vi "FastRoutineSample.vi"() -> ()   [LabVIEW 2014]
doc: "This VI demonstrates how to work with a F-712 system for fast alignment tasks.\nIn the VI menu, several fast alignment settings are accessible as well as axes control tools.\n\nThe diagram shows how to combine the driver VIs for fast alignment tasks. \n\nNote: Run XXXX_Configuration_Setup (with XXXX being the product number of your PI controller) prior to running this VI."
uses:
  C:/ProgramData/PI/LabVIEW/Low Level/General command.llb/Controller names.ctl
  FastRoutineSupportVIs/Message Cluster.ctl
  C:/ProgramData/PI/LabVIEW/Low Level/General command.llb/Global2 (Array).vi
  <vilib>/Utility/file.llb/Write To Spreadsheet File (DBL).vi
panel:
  in  "Clear Error":bool
  in  "Event timeout":i32=40
  out "3DGraphReferenceArray":refnum<vi>[](array[refnum])
  in  "Stop Motion":bool
  out "Area Scan Data":dbl[][][](array[numeric]) format="%.2f"
  out "Gradient Scan Names":string[](array[string])
  out "Analog value":dbl format="%.6f"
  in  "Analog Input":i32=1 min=1 max=10 step=1
  out "Waveform Chart":dbl(graph)
  in  "Routines Tab":T1(tab)
  in  "Area Scan Routines":T3(array[cluster]) {"Sys" min=1 step=1}
  in  "Gradient Scan Routines":T4(array[cluster]) {"Sys" min=1 step=1}
  in  "Start GS Routines":bool
  in  "Stop GS Routines":bool
  out "Controller name":T2
  in  "System no.":i32=1 min=1 step=1
  out "Status Message":string
  in  "Stop":bool
  # "This VI demonstrates how to work with a F-712 system for fast alignment tasks.\nIn the VI menu, several fast alignment settings are accessible as well as axes control tools.\n\nThe diagram shows how to combine the driver VIs for fast alignment tasks. \n\nNote:  Run XXXX_Configuration_Setup (with XXXX being the product number of your PI controller) prior to running this VI."
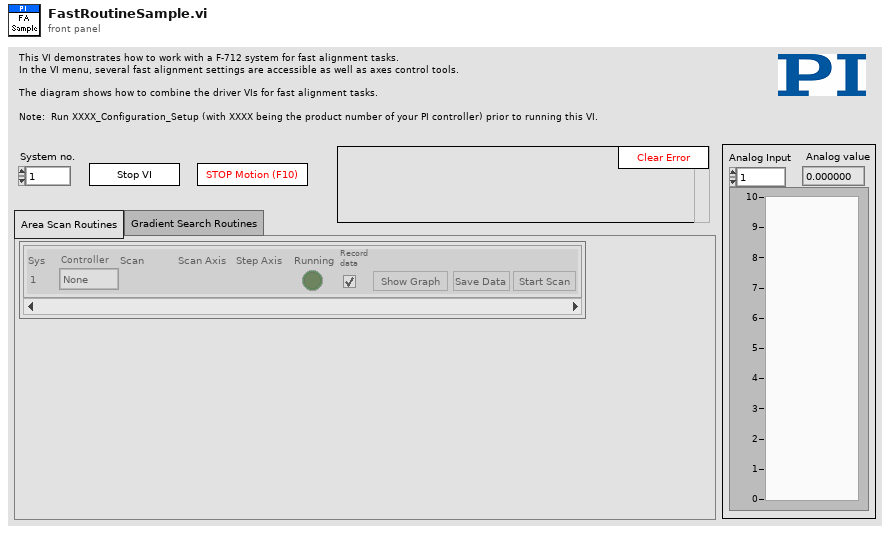
[diagram p1: front panel]
types:
  T1 = enum32{"Area Scan Routines", "Gradient Search Routines"}
  T2 = typedef "Controller names.ctl" = enum16{"None", "Analog", "C-702", "C-413", "C-414", "C-843", "C-843.PM", "C-844", "C-848", "C-865", "C-866", "C-867", "C-877", "C-880", "C-884", "C-885", "C-886", "C-887", "C-891", "E-135", "E-516", "E-517", "E-518", "E-709", "E-710", "E-712", "E-725", "E-727", "E-753", "E-754", "E-755", "E-761", "E-816", "E-861", "E-870", "E-871", "E-872", "E-873", "E-874", "F-206", "HydraPollux", "M-840", "M-850", "M-8X0", "Mercury", "Mercury_GCS", "PI_GCS2"}
  T3 = cluster{"Sys":i32, "Controller":T2, "Scan":string, "Scan Axis":string, "Step Axis":string, "Running":bool, "Record\ndata":bool, "Show Graph":bool, "Save Data":bool, "Start Scan":bool}[]
  T4 = cluster{"Sys":i32, "Scan":string, "Scan Axis":string, "Step Axis":string, "Running":bool, "Enable":bool, "Show Graph":bool, "Controller":T2, "Show Raw Data":bool}[]
  T5 = typedef "Message Cluster.ctl" = cluster{"Message":string, "Message Data":variant}
  T6 = cluster{"Sys":i32, "Scan":string, "Scan Axis":string, "Step Axis":string, "Running":bool, "Enable":bool, "Show Graph":bool, "Controller":T2, "Show Raw Data":bool}
  T7 = cluster{"Sys":i32, "Controller":T2, "Scan":string, "Scan Axis":string, "Step Axis":string, "Running":bool, "Record\ndata":bool, "Show Graph":bool, "Save Data":bool, "Start Scan":bool}
  T8 = cluster{"System No.":i32, "Scan":string, "Scan Axis":string, "Step Axis":string, "Running":bool, "Enable":bool, "Show Graph":bool, "Controller":T2, "Show Raw Data":bool}
  T9 = enum16{"open", "replace", "create", "open or create", "replace or create", "replace or create with confirmation"}
  T10 = cluster{"Gradient Scan Names":string[], "Dither Radius":dbl[], "Scan axis center":dbl[], "Step axis center":dbl[]}
  T11 = cluster{"Axis":string, "Target":dbl, "System no.":i32}
  T12 = cluster{"String to send":string, "System no.":i32}
  T13 = cluster{"Conn. axes":string[], "Controller name":T2}[]
  T14 = cluster{"Conn. axes":string[], "Controller name":T2}
  T15 = cluster{"Scan name":string, "Scan range minimum":dbl, "Scan range maximum":dbl, "Step range minimum":dbl, "Step range maximum":dbl}[]
  T16 = cluster{"Sys":i32, "Controller":T2, "Scan":string, "Successful":bool, "Signal Intensity at max":dbl, "Positions at max.":string, "Duration (s)":dbl}[]
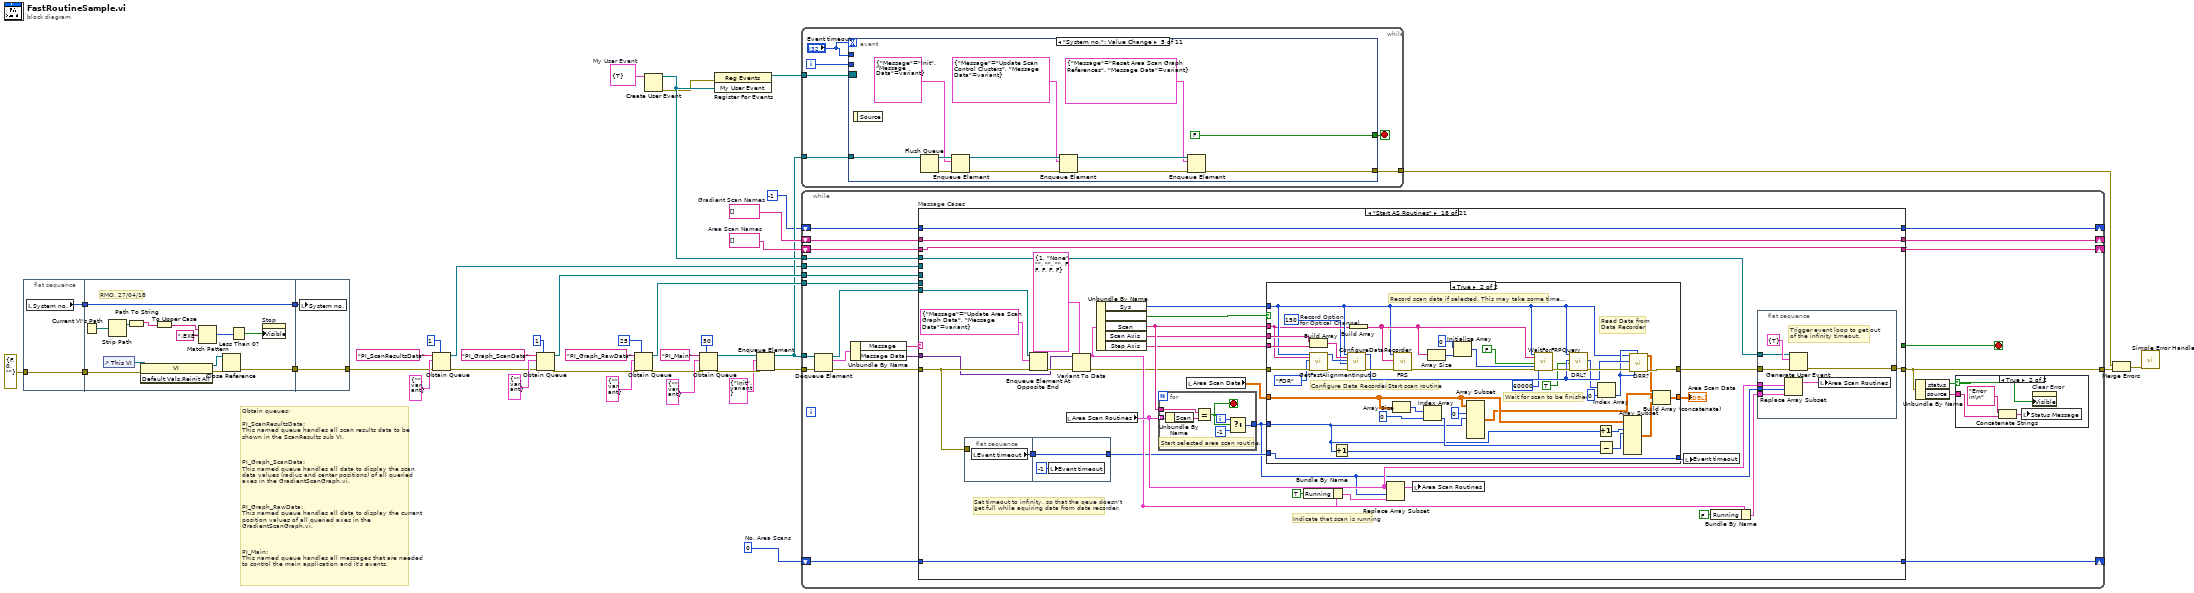
[diagram p0: block diagram]
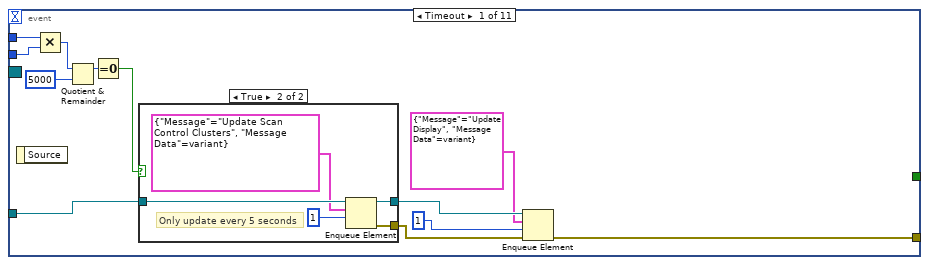
[diagram p2: hidden frame]
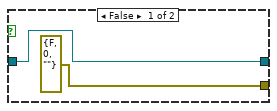
[diagram p3: hidden frame]
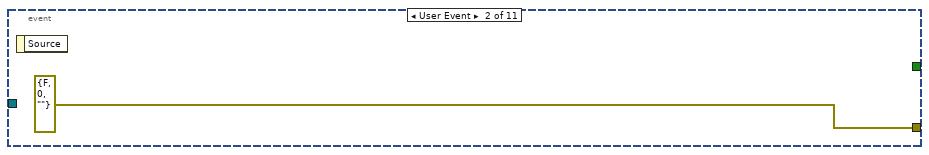
[diagram p4: hidden frame]
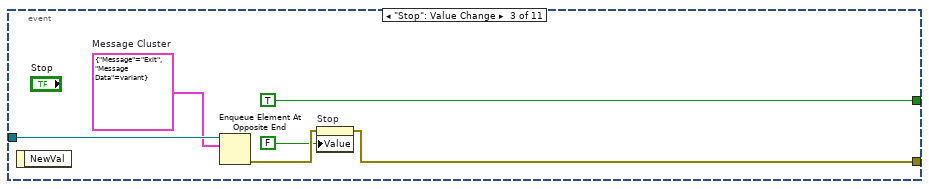
[diagram p5: hidden frame]
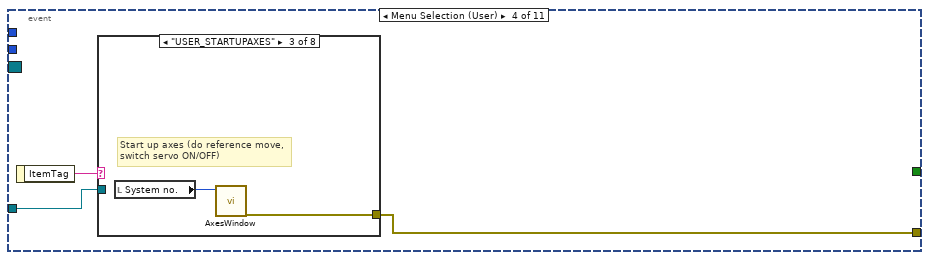
[diagram p6: hidden frame]
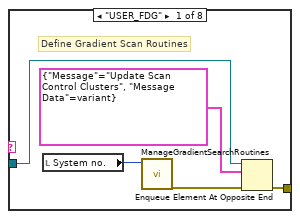
[diagram p7: hidden frame]
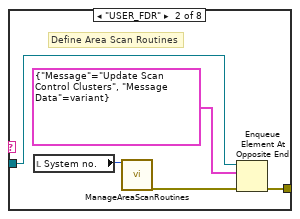
[diagram p8: hidden frame]
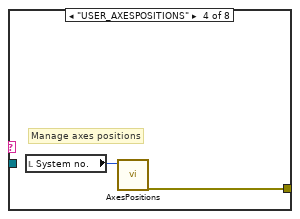
[diagram p9: hidden frame]
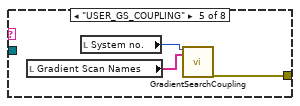
[diagram p10: hidden frame]
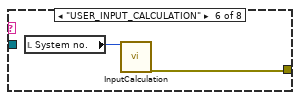
[diagram p11: hidden frame]
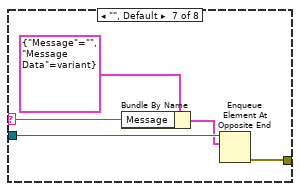
[diagram p12: hidden frame]
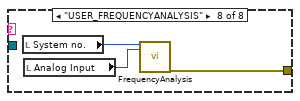
[diagram p13: hidden frame]
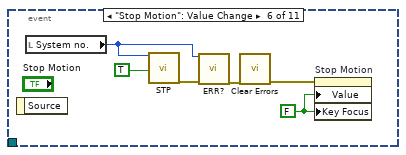
[diagram p14: hidden frame]
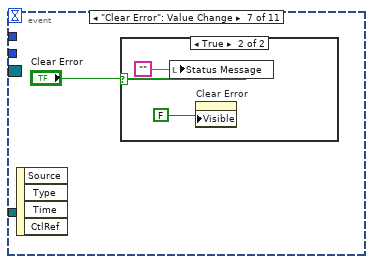
[diagram p15: hidden frame]
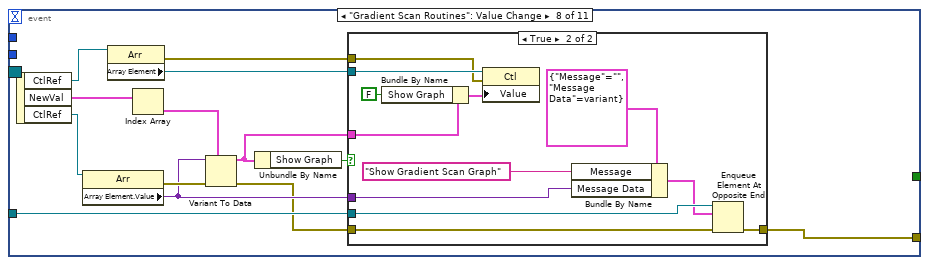
[diagram p17: hidden frame]
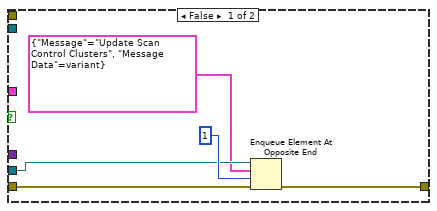
[diagram p18: hidden frame]
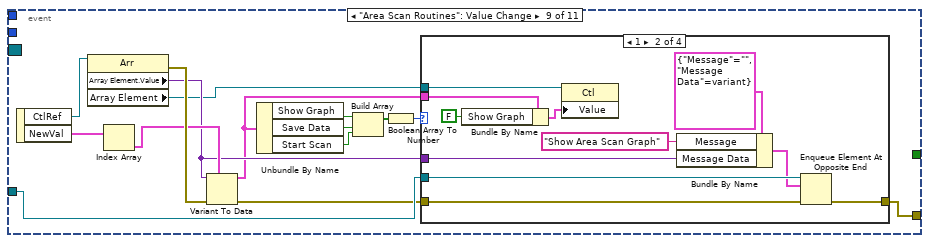
[diagram p19: hidden frame]
diagram:
  w8 = cluster{"Trigger":bool} {"Trigger"=TRUE}  # My User Event
  w20 = 0  # No. Area Scans
  w22 = string[] []  # Area Scan Names
  w23 = string[] []  # Gradient Scan Names
  # "Obtain queues:\n\nPI_ScanResultsData:\nThis named queue handles all scan results data to be shown in the ScanResults sub VI.\n\n\n\nPI_Graph_ScanData:\nThis named queue handles all data to display the scan data values (radius and center positions) of all queried axes in the GradientScanGraph.vi. \n\n\n\nPI_Graph_RawData:\nThis named queue handles all data to display the current position values of all queried axes in the GradientScanGraph.vi. \n\n\n\nPI_Main:\nThis named queue handles all messages that are needed to control the main application and it's events."
  n1 = flat-sequence {
    tunnel: errorcluster {"status"=FALSE, "code"=0, "source"=""} ("error in (no error)") -> [w42]
    tunnel: [w42] -> w3
    tunnel: [w41] -> w1
    tunnel: [w52] -> w4
    tunnel: w3 -> [w51]
    tunnel: [w50] -> w2
    tunnel: w1 -> [w50]
    tunnel: [w57] -> w11
    tunnel: w4 -> [w57]
    tunnel: w2 -> [w56]
    frame #0 {
      n2 = local read "System no."() -> (w41:i32)
    }
    frame #1 {
      # "RMO, 27/04/18"
      n3 = Current VI's Path() -> (path=w44:path)
      n4 = control-ref of="This VI"() -> (w55:refnum<vi>)
      n5 = Strip Path(path=w44) -> (stripped path=w45:path)  [unwired: 1 out]
      n6 = Path To String(path=w45) -> (string=w46:string)
      n7 = invoke class="VI" method="Default Vals.Reinit All"(reference=w55, error in=w51) -> (reference out=w54:refnum<vi>, error out=w53:errorcluster)  [unwired: 1 in, 1 out]
      n8 = To Upper Case(1:w46) -> (0:w47:string)
      n9 = Match Pattern(string=w47, regular expression=".EXE") -> (offset past match=w49:i32)  [unwired: 4 out]
      n10 = Close Reference(reference=w54, error in (no error)=w53) -> (error out=w52:errorcluster)
      n11 = Less Than 0?(x=w49) -> (x < 0?=w43:bool)
      n12 = property on="Stop" class="Bool (strict)"("Visible"=w43) -> ()  [unwired: 2 in, 2 out]
    }
    frame #2 {
      n13 = local write "System no."(w56) -> ()
    }
  }
  n14 = Obtain Queue(max queue size (-1, unlimited)=1, name (unnamed)="PI_ScanResultsData", element data type=T5 {"Message"="", "Message Data"=variant} ("Message Cluster"), error in (no error)=w11) -> (queue out=w10:refnum<queue>, error out=w12:errorcluster)  [unwired: 1 in, 1 out]
  n15 = Obtain Queue(max queue size (-1, unlimited)=1, name (unnamed)="PI_Graph_ScanData", element data type=T5 {"Message"="", "Message Data"=variant} ("Message Cluster"), error in (no error)=w12) -> (queue out=w24:refnum<queue>, error out=w25:errorcluster)  [unwired: 1 in, 1 out]
  n16 = Obtain Queue(max queue size (-1, unlimited)=25, name (unnamed)="PI_Graph_RawData", element data type=T5 {"Message"="", "Message Data"=variant} ("Message Cluster"), error in (no error)=w25) -> (queue out=w30:refnum<queue>, error out=w19:errorcluster)  [unwired: 1 in, 1 out]
  n17 = Create User Event(user event datatype=w8) -> (user event=w40:refnum<user-event>, error out=w9:errorcluster)  [unwired: 1 in]
  n18 = Obtain Queue(max queue size (-1, unlimited)=50, name (unnamed)="PI_Main", element data type=T5 {"Message"="", "Message Data"=variant} ("Message Cluster"), error in (no error)=w19) -> (queue out=w37:refnum<queue>, error out=w38:errorcluster)  [unwired: 1 in, 1 out]
  n19 = register-events(error in=w9, w40) -> (reference out=w7:refnum<event-registration>)  [unwired: 1 in, 1 out]
  n20 = Enqueue Element(queue=w37, element=T5 {"Message"="Init", "Message Data"=variant}, error in (no error)=w38) -> (queue out=w21:refnum<queue>, error out=w36:errorcluster)  [unwired: 2 out]
  n21 = while {
    tunnel: w21 -> [w63]
    tunnel: [w61] -> w18
    tunnel: w7 -> [w59]
    i -> [w60]
    stop <- w62 stop-if-true
    n22 = event shown="[4] \"System no.\": Value Change" {
      selector: w59 -> [_ _ _ _ _ _ _ _ _ _ _]
      dyn-events: _ -> [_ _ _ _ _ _ _ _ _ _ _]
      timeout: "Event timeout" -> [_ _ _ _ _ _ _ _ _ _ _]
      tunnel: [_ _ TRUE _ FALSE _ _ _ _ _ _] -> w62
      tunnel: w63 -> [w68 _ w89 w90 w130 _ _ w153 w185 w224 w231]
      tunnel: [w71 errorcluster {"status"=FALSE, "code"=0, "source"=""} ("error out") w86 w91 w123 _ _ w152 w184 w225 w226] -> w61
      tunnel: w60 -> [w66 _ _ _ _ _ _ _ _ _ _]
      tunnel: "Event timeout" -> [w67 _ _ _ _ _ _ _ _ _ _]
      event Timeout {
        n23 = event-data() -> ()  [unwired: 2 out]
        n24 = Multiply(x=w67, y=w66) -> (x*y=w65:i32)
        n25 = Quotient & Remainder(x=w65, y=5000) -> (x-y*floor(x/y)=w74:i32)  [unwired: 1 out]
        n26 = Equal To 0?(x=w74) -> (x = 0?=w73:bool)
        n27 = case shown="True" w73 {
          tunnel: [errorcluster {"status"=FALSE, "code"=0, "source"=""} ("error out") w82] -> w70
          tunnel: w68 -> [w76 w81]
          tunnel: [w76 w79] -> w69
          frame False {
          }
          frame True {
            # "Only update every 5 seconds"
            n28 = Enqueue Element(queue=w81, element=T5 {"Message"="Update Scan Control Clusters", "Message Data"=variant} ("Message Cluster"), timeout in ms (-1)=1) -> (queue out=w79:refnum<queue>, error out=w82:errorcluster)  [unwired: 1 in, 1 out]
          }
        }
        n29 = Enqueue Element(queue=w69, element=T5 {"Message"="Update Display", "Message Data"=variant} ("Message"), timeout in ms (-1)=1, error in (no error)=w70) -> (error out=w71:errorcluster)  [unwired: 2 out]
      }
      event User Event {
        n30 = event-data() -> ()  [unwired: 2 out]
      }
      event "Stop": Value Change {
        w84 = T5 {"Message"="Exit", "Message Data"=variant}  # Message Cluster
        n31 = event-data() -> ()  [unwired: 2 out]
        n32 = Enqueue Element At Opposite End(queue=w89, element=w84) -> (error out=w87:errorcluster)  [unwired: 1 in, 3 out]
        n33 = property on="Stop" class="Bool (strict)"(error in=w87, "Value"=FALSE) -> (error out=w86:errorcluster)  [unwired: 1 in, 1 out]
      }
      event Menu Selection (User) {
        n34 = event-data() -> ("ItemTag"=w92:string)  [unwired: 1 out]
        n35 = case shown="\"USER_STARTUPAXES\"" w92 {
          selector: w92 -> [_ _ _ _ _ _ w113 _]
          tunnel: [w96 w99 w104 w106 w109 w111 w116 w119] -> w91
          tunnel: w90 -> [w95 w100 _ _ _ _ w115 _]
          frame "USER_FDG" {
            # "Define Gradient Scan Routines"
            n36 = local read "System no."() -> (w93:i32)
            n37 = call "ManageGradientSearchRoutines.vi"("System no."=w93) -> ("error out"=w97:errorcluster)  [unwired: 1 in, 17 out]
            n38 = Enqueue Element At Opposite End(queue=w95, element=T5 {"Message"="Update Scan Control Clusters", "Message Data"=variant} ("Message Cluster"), error in (no error)=w97) -> (error out=w96:errorcluster)  [unwired: 3 out]
          }
          frame "USER_FDR" {
            # "Define Area Scan Routines"
            n39 = local read "System no."() -> (w98:i32)
            n40 = call "ManageAreaScanRoutines.vi"("System no."=w98) -> ("error out"=w101:errorcluster)  [unwired: 1 in, 17 out]
            n41 = Enqueue Element At Opposite End(queue=w100, element=T5 {"Message"="Update Scan Control Clusters", "Message Data"=variant} ("Message Cluster"), error in (no error)=w101) -> (error out=w99:errorcluster)  [unwired: 3 out]
          }
          frame "USER_STARTUPAXES" {
            # "Start up axes (do reference move, \nswitch servo ON/OFF)"
            n42 = local read "System no."() -> (w103:i32)
            n43 = call "AxesWindow.vi"("System no."=w103) -> ("error out"=w104:errorcluster)  [unwired: 1 in, 17 out]
          }
          frame "USER_AXESPOSITIONS" {
            # "Manage axes positions"
            n44 = local read "System no."() -> (w105:i32)
            n45 = call "AxesPositions.vi"("System no."=w105) -> ("error out"=w106:errorcluster)  [unwired: 1 in, 17 out]
          }
          frame "USER_GS_COUPLING" {
            n46 = local read "Gradient Scan Names"() -> (w108:string[])
            n47 = local read "System no."() -> (w107:i32)
            n48 = call "GradientSearchCoupling.vi"("System no."=w107, "Gradient Scan Names"=w108) -> ("error out"=w109:errorcluster)  [unwired: 1 in, 16 out]
          }
          frame "USER_INPUT_CALCULATION" {
            n49 = local read "System no."() -> (w110:i32)
            n50 = call "InputCalculation.vi"("System no."=w110) -> ("error out"=w111:errorcluster)  [unwired: 1 in, 17 out]
          }
          frame "", Default {
            n51 = Bundle By Name(cluster=T5 {"Message"="", "Message Data"=variant} ("Message"), "Message"=w113) -> (w112:T5)
            n52 = Enqueue Element At Opposite End(queue=w115, element=w112) -> (error out=w116:errorcluster)  [unwired: 1 in, 3 out]
          }
          frame "USER_FREQUENCYANALYSIS" {
            n53 = local read "System no."() -> (w118:i32)
            n54 = local read "Analog Input"() -> (w117:i32)
            n55 = call "FrequencyAnalysis.vi"("System no."=w118, "Analog Input Channel"=w117) -> ("error out"=w119:errorcluster)  [unwired: 1 in, 16 out]
          }
        }
      }
      event "System no.": Value Change {
        n56 = event-data() -> ()  [unwired: 2 out]
        n57 = Flush Queue(queue=w130) -> (queue out=w128:refnum<queue>, error out=w129:errorcluster)  [unwired: 1 in, 1 out]
        n58 = Enqueue Element(queue=w128, element=T5 {"Message"="Init", "Message Data"=variant} ("Message"), error in (no error)=w129) -> (queue out=w127:refnum<queue>, error out=w126:errorcluster)  [unwired: 2 out]
        n59 = Enqueue Element(queue=w127, element=T5 {"Message"="Update Scan Control Clusters", "Message Data"=variant} ("Message"), error in (no error)=w126) -> (queue out=w124:refnum<queue>, error out=w125:errorcluster)  [unwired: 2 out]
        n60 = Enqueue Element(queue=w124, element=T5 {"Message"="Reset Area Scan Graph References", "Message Data"=variant} ("Message"), error in (no error)=w125) -> (error out=w123:errorcluster)  [unwired: 3 out]
      }
      event "Stop Motion": Value Change {
        w132 = FALSE
        n61 = event-data() -> ()  [unwired: 2 out]
        n62 = local read "System no."() -> (w135:i32)
        n63 = call "STP.vi"("System no."=w135, "All axes?"=TRUE) -> ("error out"=w136:errorcluster)  [unwired: 3 in, 14 out]
        n64 = call "ERR?.vi"("System no."=w135, "error in"=w136) -> ("error out"=w134:errorcluster)  [unwired: 17 out]
        n65 = call <vilib>:"Clear Errors.vi"("error in (no error)"=w134) -> ("error out"=w133:errorcluster)  [unwired: 1 in, 5 out]
        n66 = property on="Stop Motion" class="Bool"(error in=w133, "Value"=w132, "Key Focus"=w132) -> ()  [unwired: 1 in, 2 out]
      }
      event "Clear Error": Value Change {
        n67 = event-data() -> ()  [unwired: 5 out]
        n68 = case shown="True" "Clear Error" {
          frame False {
          }
          frame True {
            n69 = local write "Status Message"("") -> ()
            n70 = property on="Clear Error" class="Bool"("Visible"=FALSE) -> ()  [unwired: 2 in, 2 out]
          }
        }
      }
      event "Gradient Scan Routines": Value Change {
        n71 = event-data() -> ("CtlRef"=w143:refnum<vi>, "NewVal"=w149:T4, "CtlRef"=w144:refnum<vi>)  [unwired: 1 out]
        n72 = property class="Arr"(reference=w144) -> (error out=w151:errorcluster, "Array Element.Value"=w148:variant)  [unwired: 1 in, 1 out]
        n73 = property class="Arr"(reference=w143) -> (error out=w141:errorcluster, "Array Element"=w142:refnum<vi>)  [unwired: 1 in, 1 out]
        n74 = Index Array(array=w149) -> (element=w150:T6)  [unwired: 1 in]
        n75 = Variant To Data(error in=w151, type=w150, Variant=w148) -> (data=w145:T6, error out=w147:errorcluster)
        n76 = Unbundle By Name(w145) -> ("Show Graph"=w146:bool)
        n77 = case shown="True" w146 {
          tunnel: w153 -> [w155 w170]
          tunnel: [w156 w169] -> w152
          tunnel: w148 -> [_ w166]
          tunnel: w147 -> [w157 w165]
          tunnel: w142 -> [_ w162]
          tunnel: w145 -> [_ w161]
          tunnel: w141 -> [_ w159]
          frame False {
            n78 = Enqueue Element At Opposite End(queue=w155, element=T5 {"Message"="Update Scan Control Clusters", "Message Data"=variant} ("Message"), timeout in ms (-1)=1, error in (no error)=w157) -> (error out=w156:errorcluster)  [unwired: 2 out]
          }
          frame True {
            n79 = Bundle By Name(cluster=w161, "Show Graph"=FALSE) -> (w163:T6)
            n80 = property class="Ctl"(reference=w162, error in=w159, "Value"=w163) -> ()  [unwired: 2 out]
            n81 = Bundle By Name(cluster=T5 {"Message"="", "Message Data"=variant} ("Message"), "Message"="Show Gradient Scan Graph", "Message Data"=w166) -> (w168:T5)
            n82 = Enqueue Element At Opposite End(queue=w170, element=w168, error in (no error)=w165) -> (error out=w169:errorcluster)  [unwired: 3 out]
          }
        }
      }
      event "Area Scan Routines": Value Change {
        n83 = event-data() -> ("CtlRef"=w171:refnum<vi>, "NewVal"=w177:T3)  [unwired: 1 out]
        n84 = property class="Arr"(reference=w171) -> (error out=w183:errorcluster, "Array Element.Value"=w181:variant, "Array Element"=w179:refnum<vi>)  [unwired: 1 in, 1 out]
        n85 = Index Array(array=w177) -> (element=w182:T7)  [unwired: 1 in]
        n86 = Variant To Data(error in=w183, type=w182, Variant=w181) -> (data=w178:T7, error out=w180:errorcluster)
        n87 = Unbundle By Name(w178) -> ("Show Graph"=w176:bool, "Save Data"=w175:bool, "Start Scan"=w172:bool)
        n88 = Build Array(w176, w175, w172) -> (w174:bool[])
        n89 = Boolean Array To Number(Boolean array=w174) -> (number=w173:u32)
        n90 = case shown="1" w173 {
          tunnel: w185 -> [_ w197 w208 w219]
          tunnel: [w186 w196 w207 w218] -> w184
          tunnel: w181 -> [_ w193 w199 _]
          tunnel: w180 -> [w186 w192 w204 w211]
          tunnel: w179 -> [_ w189 w201 w213]
          tunnel: w178 -> [_ w188 w200 w212]
          frame 0, Default {
          }
          frame 1 {
            n91 = Bundle By Name(cluster=w188, "Show Graph"=FALSE) -> (w190:T7)
            n92 = property class="Ctl"(reference=w189, "Value"=w190) -> ()  [unwired: 1 in, 2 out]
            n93 = Bundle By Name(cluster=T5 {"Message"="", "Message Data"=variant} ("Message"), "Message"="Show Area Scan Graph", "Message Data"=w193) -> (w195:T5)
            n94 = Enqueue Element At Opposite End(queue=w197, element=w195, error in (no error)=w192) -> (error out=w196:errorcluster)  [unwired: 3 out]
          }
          frame 2 {
            n95 = Bundle By Name(cluster=w200, "Save Data"=FALSE) -> (w202:T7)
            n96 = property class="Ctl"(reference=w201, "Value"=w202) -> ()  [unwired: 1 in, 2 out]
            n97 = Bundle By Name(cluster=T5 {"Message"="", "Message Data"=variant} ("Message"), "Message"="Save Area Scan Data", "Message Data"=w199) -> (w206:T5)
            n98 = Enqueue Element At Opposite End(queue=w208, element=w206, error in (no error)=w204) -> (error out=w207:errorcluster)  [unwired: 3 out]
          }
          frame 4 {
            n99 = Bundle By Name(cluster=w212, "Start Scan"=FALSE) -> (w214:T7)
            n100 = property class="Ctl"(reference=w213, "Value"=w214) -> ("Value"=w209:variant)  [unwired: 1 in, 2 out]
            n101 = Bundle By Name(cluster=T5 {"Message"="", "Message Data"=variant} ("Message"), "Message"="Start AS Routines", "Message Data"=w209) -> (w217:T5)
            n102 = Enqueue Element At Opposite End(queue=w219, element=w217, error in (no error)=w211) -> (error out=w218:errorcluster)  [unwired: 3 out]
          }
        }
      }
      event "Start GS Routines": Value Change {
        w220 = T5 {"Message"="", "Message Data"=variant}  # Message Cluster
        n103 = event-data() -> ("CtlRef"=w223:refnum<vi>)  [unwired: 1 out]
        n104 = property class="Bool"(reference=w223) -> ("Label.Text"=w222:string)  [unwired: 1 in, 2 out]
        n105 = Bundle By Name(cluster=w220, "Message"=w222) -> (w221:T5)
        n106 = Enqueue Element At Opposite End(queue=w224, element=w221) -> (error out=w225:errorcluster)  [unwired: 1 in, 3 out]
      }
      event "Stop GS Routines": Value Change {
        w227 = T5 {"Message"="", "Message Data"=variant}  # Message Cluster
        n107 = event-data() -> ("CtlRef"=w230:refnum<vi>)  [unwired: 1 out]
        n108 = property class="Bool"(reference=w230) -> ("Label.Text"=w229:string)  [unwired: 1 in, 2 out]
        n109 = Bundle By Name(cluster=w227, "Message"=w229) -> (w228:T5)
        n110 = Enqueue Element At Opposite End(queue=w231, element=w228) -> (error out=w226:errorcluster)  [unwired: 1 in, 3 out]
      }
    }
  }
  n111 = while {
    tunnel: w21 -> [w252]
    tunnel: w30 -> [w246]
    tunnel: w24 -> [w245]
    shift-right: [w244] -> _
    shift-left: w23 -> [w243]
    shift-right: [w241] -> _
    shift-left: w22 -> [w242]
    shift-right: [w240] -> _
    shift-left: -1 ("System no.") -> [w239]
    shift-right: [w237] -> _
    shift-left: w20 -> [w238]
    tunnel: w10 -> [w236]
    tunnel: w36 -> [w253]
    tunnel: [w235] -> w17
    tunnel: w40 -> [w232]
    stop <- w254 stop-if-true
    n112 = Dequeue Element(queue=w252, error in (no error)=w253) -> (queue out=w250:refnum<queue>, element=w251:T5, error out=w249:errorcluster)  [unwired: 2 out]
    n113 = Unbundle By Name(w251) -> ("Message"=w248:string, "Message Data"=w247:variant)
    n114 = case "Message Cases" shown="\"Start AS Routines\"" w248 {
      tunnel: w250 -> [w261 _ _ _ _ _ _ _ w608 _ _ w732 _ _ _ w890 _ w960 _ w1083 _]
      tunnel: w249 -> [w272 w308 w324 w354 w418 w485 w517 w567 w612 w630 w665 w750 w815 w873 w887 w902 w925 w961 w1051 w1082 w1094]
      tunnel: [w263 w305 w323 w352 w421 w461 w509 w555 w607 w631 w666 w753 w817 w861 w876 w891 w925 w938 w1052 w1068 w1094] -> w235
      tunnel: [w262 _ _ _ _ _ _ _ _ _ _ _ _ _ _ _ _ _ _ TRUE _] -> w254
      tunnel: w247 -> [_ _ _ _ w419 w484 w516 w566 _ _ _ _ w813 w871 w886 _ _ w958 _ _ _]
      tunnel: w246 -> [_ _ _ _ _ _ _ _ _ _ _ w760 _ _ _ _ _ _ _ _ _]
      tunnel: w245 -> [_ _ _ _ _ _ _ _ _ _ _ w721 _ _ _ _ _ _ _ w1073 _]
      tunnel: [w270 w316 w335 w381 w397 w489 w505 w572 w616 w635 w661 w718 w810 w869 w884 w900 w929 w968 w1046 w1078 w1093] -> w244
      tunnel: w243 -> [_ w316 w335 w381 w397 w489 w505 w572 w616 w635 _ w718 w810 w869 w884 w900 w929 w968 w1046 w1078 w1093]
      tunnel: w242 -> [_ w315 w334 w380 w396 w486 w518 w571 w606 w634 _ w729 w809 w868 w883 w899 w928 w967 w1045 w1077 w1092]
      tunnel: [w271 w315 w334 w380 w396 w486 w518 w571 w606 w634 w675 w729 w809 w868 w883 w899 w928 w967 w1045 w1077 w1092] -> w241
      tunnel: ["System no." w314 w333 w353 w395 w488 w520 w556 w615 w628 w660 w731 w808 w867 w879 w898 w927 w954 w1044 w1076 w1091] -> w240
      tunnel: w239 -> [w260 w314 w333 w353 w395 w488 w520 w556 w615 w628 w660 w731 w808 w867 w879 w898 w927 w954 w1044 w1076 w1091]
      tunnel: w238 -> [w275 w313 w332 w379 w394 w479 w515 w570 _ w633 w676 w733 w801 w864 w882 w896 w926 w964 w1042 w1075 w1090]
      tunnel: [w275 w313 w332 w379 w394 w479 w515 w570 w614 w633 w676 w734 w801 w864 w882 w896 w926 w964 w1042 w1075 w1090] -> w237
      tunnel: w236 -> [_ _ _ _ _ _ _ _ _ _ _ w726 _ _ _ _ _ _ _ w1070 _]
      tunnel: w232 -> [_ _ _ _ _ _ _ _ _ _ _ _ _ _ _ _ _ w942 _ _ _]
      frame "Init" {
        w271 = string[] []  # Area Scan Names
        w270 = string[] []  # Gradient Scan Names
        w259 = "Connected to:\n"
        # "Query identification of connected controller."
        n115 = call "*IDN?.vi"("System no."="System no.", "error in"=w272) -> ("Identification"=w274:string, "error out"=w264:errorcluster)  [unwired: 16 out]
        n116 = Concatenate Strings(w259, w274) -> (→"Status Message":string)
        n117 = call "ERR?.vi"("error in"=w264) -> ("Controller error"=w267:bool, "error out"=w269:errorcluster)  [unwired: 1 in, 16 out]
        n118 = Unbundle By Name(w269) -> ("status"=w268:bool)
        n119 = Not(x=w267) -> (.not. x?=w266:bool)
        n120 = And(x=w266, y=w268) -> (x .and. y?=w265:bool)
        n121 = case shown="True" w265 {
          tunnel: [w282 w290] -> w263
          tunnel: w261 -> [w281 w291]
          tunnel: [FALSE w292] -> w262
          tunnel: w260 -> [_ w287]
          tunnel: w269 -> [w279 w285]
          tunnel: w259 -> [_ w283]
          frame False {
            n122 = call <vilib>:"Clear Errors.vi"("error in (no error)"=w279) -> ("error out"=w278:errorcluster)  [unwired: 1 in, 5 out]
            n123 = Enqueue Element At Opposite End(queue=w281, element=T5 {"Message"="Show ScanResults Window", "Message Data"=variant} ("Message Cluster"), error in (no error)=w278) -> (error out=w282:errorcluster)  [unwired: 3 out]
          }
          frame True {
            n124 = call <vilib>:"Clear Errors.vi"("error in (no error)"=w285) -> ("error out"=w289:errorcluster)  [unwired: 1 in, 5 out]
            n125 = call "*IDN?.vi"("System no."=w287, "error in"=w289) -> ("Identification"=w286:string, "error out"=w284:errorcluster)  [unwired: 16 out]
            n126 = Concatenate Strings(w283, w286) -> (w288:string)
            n127 = local write "Status Message"(w288) -> ()
            n128 = case shown="Error" w284 {
              selector: w284 -> [w294 w297]
              tunnel: [FALSE TRUE] -> w292
              tunnel: w291 -> [_ w303]
              tunnel: [w293 w299] -> w290
              tunnel: w287 -> [w295 _]
              frame No Error {
                # "If previous system number works, \nthen switch back to previous number."
                n129 = property on="System no." class="DigNum (strict)"(error in=w294, "Val(Sgnl)"=w295, "Value"=w295) -> (error out=w293:errorcluster)  [unwired: 1 in, 1 out]
              }
              frame Error {
                # "If *IDN? reports an error,\nthe system is probably not connected."
                n130 = property on="Stop" class="Bool (strict)"("Val(Sgnl)"=TRUE) -> (error out=w300:errorcluster)  [unwired: 2 in, 1 out]
                n131 = Enqueue Element At Opposite End(queue=w303, element=T5 {"Message"="Exit", "Message Data"=variant}, error in (no error)=w300) -> (error out=w298:errorcluster)  [unwired: 3 out]
                n132 = Merge Errors(w297, w298) -> (w299:errorcluster)
              }
            }
          }
        }
      }
      frame "USER_AXESCONTROL" {
        # "Show Axes Control window."
        n133 = vi-ref "AxesControl.vi"() -> (w318:refnum<vi>)
        n134 = property class="VI"(reference=w318, error in=w308) -> (error out=w307:errorcluster, "Path"=w319:path)  [unwired: 1 out]
        n135 = Open VI Reference(vi path=w319, options=8, error in (no error)=w307) -> (vi reference=w317:refnum<vi>, error out=w306:errorcluster)  [unwired: 1 in, 2 out]
        n136 = property class="VI"(reference=w317, error in=w306, "Front Panel.Open"=TRUE ("Front Panel Window:Open")) -> (reference out=w309:refnum<vi>, error out=w310:errorcluster)
        n137 = invoke class="VI" method="Run VI"(reference=w309, error in=w310, "Wait until done"=FALSE ("Front Panel Window:Open"), "Auto Dispose Ref"=TRUE ("Front Panel Window:Open")) -> (error out=w305:errorcluster)  [unwired: 1 in, 4 out]
      }
      frame "USER_TERMINAL" {
        # "Show Terminal window."
        n138 = vi-ref "PITerm.vi"() -> (w322:refnum<vi>)
        n139 = property class="VI"(reference=w322, error in=w324) -> (error out=w330:errorcluster, "Path"=w331:path)  [unwired: 1 out]
        n140 = Open VI Reference(vi path=w331, error in (no error)=w330) -> (vi reference=w325:refnum<vi>, error out=w326:errorcluster)  [unwired: 1 in, 3 out]
        n141 = property class="VI"(reference=w325, error in=w326) -> (reference out=w328:refnum<vi>, error out=w329:errorcluster, "Front Panel.Open"=w327:bool)
        n142 = case shown="False" w327 {
          tunnel: w329 -> [w339 w344]
          tunnel: w328 -> [w338 _]
          tunnel: [w336 w344] -> w323
          frame False {
            n143 = property class="VI"(reference=w338, error in=w339, "Front Panel.Open"=TRUE ("Front Panel Window:Open")) -> (reference out=w340:refnum<vi>, error out=w341:errorcluster)
            n144 = invoke class="VI" method="Run VI"(reference=w340, error in=w341, "Wait until done"=FALSE ("Wait Until Done"), "Auto Dispose Ref"=TRUE ("Front Panel Window:Open")) -> (error out=w336:errorcluster)  [unwired: 1 in, 4 out]
          }
          frame True {
          }
        }
      }
      frame "USER_POSITIONGRAPH" {
        n145 = global read "Global2 (Array).vi" "System"() -> (w376:T13)
        n146 = Decrement(x=w353) -> (x-1=w375:i32)
        n147 = vi-ref "GradientSearchGraph.vi"() -> (w371:refnum<vi>)
        n148 = Index Array(array=w376, index=w375) -> (element=w374:T14)
        n149 = property class="VI"(reference=w371, error in=w354) -> (error out=w370:errorcluster, "Path"=w372:path)  [unwired: 1 out]
        n150 = Unbundle By Name(w374) -> ("Controller name"=w365:T2)
        n151 = Open VI Reference(vi path=w372, options=8, error in (no error)=w370) -> (vi reference=w369:refnum<vi>, error out=w368:errorcluster)  [unwired: 1 in, 2 out]
        n152 = flat-sequence {
          tunnel: w365 -> [w383]
          tunnel: [w382] -> w363
          frame #0 {
            n153 = property on="Controller name" class="Enum (strict)"() -> ("Strings []"=w384:string[])  [unwired: 2 in, 2 out]
            n154 = Index Array(array=w384, index=w383) -> (element=w382:string)
          }
        }
        n155 = property class="VI"(reference=w369, error in=w368, "Front Panel.Open"=TRUE ("Front Panel Window:Open")) -> (reference out=w359:refnum<vi>, error out=w358:errorcluster)
        n156 = invoke class="VI" method="Ctrl Val.Set"(reference=w359, error in=w358, "Control Name"="System no.", "Value"=w353) -> (reference out=w347:refnum<vi>, error out=w350:errorcluster)  [unwired: 1 in, 3 out]
        n157 = Concatenate Strings(" (", w363, ")") -> (w361:string)
        n158 = Number To Decimal String(number=w353) -> (decimal integer string=w367:string)  [unwired: 1 out]
        n159 = Concatenate Strings("System ", w367, w361) -> (w360:string)
        n160 = invoke class="VI" method="Ctrl Val.Set"(reference=w347, error in=w350, "Control Name"="OverrideClone", "Value"=TRUE) -> (reference out=w348:refnum<vi>, error out=w349:errorcluster)  [unwired: 1 in, 3 out]
        n161 = property class="VI"(reference=w348, error in=w349, "Front Panel.Title"=w360) -> (reference out=w355:refnum<vi>, error out=w356:errorcluster)
        n162 = invoke class="VI" method="Run VI"(reference=w355, error in=w356, "Wait until done"=FALSE ("Wait Until Done"), "Auto Dispose Ref"=TRUE ("Front Panel Window:Open")) -> (error out=w352:errorcluster)  [unwired: 1 in, 4 out]
      }
      frame "Show Gradient Scan Graph" {
        # "Open gradient scan routine graph."
        n163 = Variant To Data(error in=w418, type=T8 {"System No."=0, "Scan"="", "Scan Axis"="", "Step Axis"="", "Running"=FALSE, "Enable"=FALSE, "Show Graph"=FALSE, "Controller"=enum."None", "Show Raw Data"=FALSE} ("element"), Variant=w419) -> (data=w417:T8, error out=w415:errorcluster)
        n164 = Unbundle By Name(w417) -> ("Step Axis"=w385:string, "Scan Axis"=w390:string, "System No."=w391:i32, "Scan"=w387:string, "Show Raw Data"=w386:bool)
        n165 = Decrement(x=w391) -> (x-1=w441:i32)
        n166 = global read "Global2 (Array).vi" "System"() -> (w442:T13)
        n167 = global read "Global2 (Array).vi" "System"() -> (w393:T13)
        n168 = vi-ref "GradientSearchGraph.vi"() -> (w432:refnum<vi>)
        n169 = property class="VI"(reference=w432, error in=w415) -> (error out=w431:errorcluster, "Path"=w433:path)  [unwired: 1 out]
        n170 = Index Array(array=w442, index=w441) -> (element=w440:T14)
        n171 = Index Array(array=w393, index=w391) -> (element=w392:T14)
        n172 = Unbundle By Name(w440) -> ("Controller name"=w414:T2)
        "Controller name" <- w414
        n173 = Unbundle By Name(w392) -> ("Conn. axes"=w388:string[])
        n174 = Open VI Reference(vi path=w433, options=8, error in (no error)=w431) -> (vi reference=w430:refnum<vi>, error out=w429:errorcluster)  [unwired: 1 in, 2 out]
        n175 = property class="VI"(reference=w430, error in=w429, "Front Panel.Open"=TRUE ("Front Panel Window:Open")) -> (reference out=w408:refnum<vi>, error out=w407:errorcluster)
        n176 = for "Get Scan Axis" {
          tunnel: w390 -> [w451]
          tunnel: w388 -> [w450] mode=indexing
          tunnel: [w446] -> w389
          i -> [w449]
          stop <- w447 stop-if-true
          n177 = Equal?(x=w451, y=w450) -> (x = y?=w447:bool)
          n178 = Select(t=w449, s=w447, f=0) -> (s? t:f=w446:i32)
        }
        n179 = for "Get Step Axis" {
          tunnel: w385 -> [w460]
          tunnel: w388 -> [w459] mode=indexing
          tunnel: [w455] -> w435
          i -> [w458]
          stop <- w456 stop-if-true
          n180 = Equal?(x=w460, y=w459) -> (x = y?=w456:bool)
          n181 = Select(t=w458, s=w456, f=0) -> (s? t:f=w455:i32)
        }
        n182 = flat-sequence {
          tunnel: w414 -> [w453]
          tunnel: [w452] -> w412
          frame #0 {
            n183 = property on="Controller name" class="Enum (strict)"() -> ("Strings []"=w454:string[])  [unwired: 2 in, 2 out]
            n184 = Index Array(array=w454, index=w453) -> (element=w452:string)
          }
        }
        n185 = invoke class="VI" method="Ctrl Val.Set"(reference=w408, error in=w407, "Control Name"="System no.", "Value"=w391) -> (reference out=w402:refnum<vi>, error out=w401:errorcluster)  [unwired: 1 in, 3 out]
        n186 = invoke class="VI" method="Ctrl Val.Set"(reference=w402, error in=w401, "Control Name"="GS Name", "Value"=w387) -> (reference out=w400:refnum<vi>, error out=w399:errorcluster)  [unwired: 1 in, 3 out]
        n187 = Concatenate Strings(" (", w412, ")") -> (w410:string)
        n188 = Number To Decimal String(number=w391) -> (decimal integer string=w426:string)  [unwired: 1 out]
        n189 = invoke class="VI" method="Ctrl Val.Set"(reference=w400, error in=w399, "Control Name"="Raw Data", "Value"=w386) -> (reference out=w405:refnum<vi>, error out=w404:errorcluster)  [unwired: 1 in, 3 out]
        n190 = Concatenate Strings("System ", w426, w410, " : ", "Gradient Search ", w387) -> (w409:string)
        n191 = property class="VI"(reference=w405, error in=w404, "Front Panel.Title"=w409) -> (reference out=w424:refnum<vi>, error out=w425:errorcluster)
        n192 = invoke class="VI" method="Ctrl Val.Set"(reference=w424, error in=w425, "Control Name"="X Axis", "Value"=w389) -> (reference out=w423:refnum<vi>, error out=w437:errorcluster)  [unwired: 1 in, 3 out]
        n193 = invoke class="VI" method="Ctrl Val.Set"(reference=w423, error in=w437, "Control Name"="Y Axis", "Value"=w435) -> (reference out=w422:refnum<vi>, error out=w436:errorcluster)  [unwired: 1 in, 3 out]
        n194 = invoke class="VI" method="Run VI"(reference=w422, error in=w436, "Wait until done"=FALSE ("Wait Until Done"), "Auto Dispose Ref"=TRUE ("Front Panel Window:Open")) -> (error out=w421:errorcluster)  [unwired: 1 in, 4 out]
      }
      frame "Show Area Scan Graph" {
        # "Open 3D graph window of corresponding area scan routine."
        n195 = Variant To Data(error in=w485, type=T7 {"Sys"=1, "Controller"=enum."None", "Scan"="", "Scan Axis"="", "Step Axis"="", "Running"=FALSE, "Record\ndata"=FALSE, "Show Graph"=FALSE, "Save Data"=FALSE, "Start Scan"=FALSE} ("GradientScans"), Variant=w484) -> (data=w487:T7, error out=w483:errorcluster)
        n196 = local read "Area Scan Routines"() -> (w482:T3)
        n197 = Unbundle By Name(w487) -> ("Scan"=w481:string)
        n198 = for {
          tunnel: w482 -> [w498] mode=indexing
          tunnel: w481 -> [w499]
          tunnel: [w493] -> w480
          i -> [w494]
          stop <- w495 stop-if-true
          n199 = Unbundle By Name(w498) -> ("Scan"=w497:string)
          n200 = Equal?(x=w497, y=w499) -> (x = y?=w495:bool)
          n201 = Select(t=w494, s=w495, f=-1) -> (s? t:f=w493:i32)
        }
        n202 = local read "3DGraphReferenceArray"() -> (w471:refnum<vi>[])
        n203 = local read "Area Scan Data"() -> (w470:dbl[][][])
        n204 = Index Array(array=w471, index=w480) -> (element=w467:refnum<vi>)
        n205 = invoke class="VI" method="Ctrl Val.Set"(reference=w467, error in=w483, "Control Name"="Area Scan Data", "Value"=w470) -> (reference out=w466:refnum<vi>, error out=w465:errorcluster)  [unwired: 1 in, 3 out]
        n206 = invoke class="VI" method="Ctrl Val.Set"(reference=w466, error in=w465, "Control Name"="Area Scan Data page", "Value"=w480) -> (reference out=w473:refnum<vi>, error out=w472:errorcluster)  [unwired: 1 in, 3 out]
        n207 = property class="VI"(reference=w473, error in=w472, "Front Panel.Open"=TRUE ("Front Panel Window:Open")) -> (reference out=w477:refnum<vi>, error out=w474:errorcluster)
        n208 = invoke class="VI" method="Run VI"(reference=w477, error in=w474, "Wait until done"=FALSE, "Auto Dispose Ref"=FALSE) -> (error out=w462:errorcluster)  [unwired: 1 in, 4 out]
        n209 = Unbundle By Name(w462) -> ("code"=w463:i32)
        n210 = case shown="1000" w463 {
          tunnel: w462 -> [w490 w491]
          tunnel: [w490 w492] -> w461
          frame 0, Default {
          }
          frame 1000 {
            # "Clear Error 1000\nif VI is already\nrunning"
            n211 = call <vilib>:"Clear Errors.vi"("error in (no error)"=w491) -> ("error out"=w492:errorcluster)  [unwired: 1 in, 5 out]
          }
        }
      }
      frame "Save Area Scan Data" {
        # "Save scan data to text file.\n\nThe file will contain 3 columns: Scan Axis position, Step Axis position and Intensity.\n\nNote: Only the positions of the scan rountine are recorded. To record the positions of more axes, please adapt the \"Start AS Routines\" case."
        n212 = local read "Area Scan Routines"() -> (w514:T3)
        n213 = Variant To Data(error in=w517, type=T7 {"Sys"=1, "Controller"=enum."None", "Scan"="", "Scan Axis"="", "Step Axis"="", "Running"=FALSE, "Record\ndata"=FALSE, "Show Graph"=FALSE, "Save Data"=FALSE, "Start Scan"=FALSE} ("GradientScans"), Variant=w516) -> (data=w519:T7, error out=w510:errorcluster)
        n214 = Unbundle By Name(w519) -> ("Scan"=w513:string)
        n215 = for {
          tunnel: w514 -> [w549] mode=indexing
          tunnel: w513 -> [w550]
          tunnel: [w552] -> w511
          i -> [w547]
          stop <- w551 stop-if-true
          n216 = Unbundle By Name(w549) -> ("Scan"=w548:string)
          n217 = Equal?(x=w548, y=w550) -> (x = y?=w551:bool)
          n218 = case shown="True" w551 {
            tunnel: w547 -> [_ w554]
            tunnel: [-1 w554] -> w552
            frame False {
            }
            frame True {
            }
          }
        }
        n219 = local read "Area Scan Data"() -> (w512:dbl[][][])
        n220 = Index Array(array=w512, index (dim 0)=w511) -> (element=w506:dbl[][])  [unwired: 2 in]
        n221 = for {
          tunnel: w506 -> [w539] mode=indexing
          shift-right: [w537] -> w500
          shift-left: dbl[][] [] ("subarray") -> [w538]
          n222 = Greater?(x=w539, y=dbl[] [0.0, 0.0, 0.0]) -> (0:w540:bool[])
          n223 = And Array Elements(Boolean array=w540) -> (logical AND=w541:bool)
          n224 = case shown="True" w541 {
            tunnel: w539 -> [_ w545]
            tunnel: w538 -> [w543 w546]
            tunnel: [w543 w544] -> w537
            frame False {
            }
            frame True {
              n225 = Build Array (concatenate)(w546, w545) -> (w544:dbl[][])
            }
          }
        }
        n226 = Open/Create/Replace File(error in=w510, operation (0:open)=T9."replace or create") -> (refnum out=w502:refnum<file>, cancelled=w504:bool, error out=w503:errorcluster)  [unwired: 4 out]
        n227 = case shown="False" w504 {
          tunnel: [w523 w535] -> w509
          tunnel: w503 -> [w521 w536]
          tunnel: w502 -> [w527 _]
          tunnel: w500 -> [w522 _]
          frame False {
            n228 = Write to Text File(file (use dialog)=w527, text="#Scan axis position\tStep axis position\tSignal\n", error in=w521) -> (refnum out=w526:refnum<file>, error out=w528:errorcluster)  [unwired: 2 out]
            n229 = Close File(refnum=w526, error in=w528) -> (path=w529:path, error out=w524:errorcluster)
            n230 = case shown="No Error" w524 {
              selector: w524 -> [w530 w534]
              tunnel: w529 -> [w533 _]
              tunnel: w522 -> [w531 _]
              tunnel: [w530 w534] -> w523
              frame No Error {
                n231 = call-poly <vilib>:"Write To Spreadsheet File.vi"("append to file? (new file:F)"=TRUE, "2D data"=w531, "file path (dialog if empty)"=w533) -> ()  [unwired: 3 in, 3 out]
              }
              frame Error {
              }
            }
          }
          frame True {
            n232 = call <vilib>:"Clear Errors.vi"("error in (no error)"=w536) -> ("error out"=w535:errorcluster)  [unwired: 1 in, 5 out]
          }
        }
      }
      frame "Update Area Scan Graph References" {
        # "When numer of area scan routines changes on controller, create new references for the 3D graph window."
        n233 = Variant To Data(error in=w567, type=0, Variant=w566) -> (data=w565:i32, error out=w557:errorcluster)
        n234 = for {
          N: w565 -> [_]
          tunnel: [w597] -> w569 mode=indexing
          shift-right: [w595] -> w563
          shift-left: w557 -> [w596]
          # "Create new references"
          n235 = vi-ref "AreaScan3DGraph.vi"() -> (w598:refnum<vi>)
          n236 = property class="VI"(reference=w598, error in=w596) -> (error out=w600:errorcluster, "Path"=w599:path)  [unwired: 1 out]
          n237 = Open VI Reference(vi path=w599, options=8, error in (no error)=w600) -> (vi reference=w597:refnum<vi>, error out=w595:errorcluster)  [unwired: 1 in, 2 out]
        }
        n238 = local read "3DGraphReferenceArray"() -> (w561:refnum<vi>[])
        n239 = Array Size(array=w561) -> (size(s)=w560:i32)
        n240 = Greater Than 0?(x=w560) -> (x > 0?=w559:bool)
        n241 = local read "Area Scan Routines"() -> (w558:T3)
        n242 = case shown="True" w559 {
          tunnel: w569 -> [w573 w576]
          tunnel: [w573 w575] -> w564
          tunnel: w561 -> [_ w574]
          frame False {
          }
          frame True {
            n243 = Insert Into Array(array=w574, new element=w576) -> (w575:refnum<vi>[])  [unwired: 1 in]
          }
        }
        n244 = for {
          tunnel: w564 -> [w591] mode=indexing
          tunnel: w558 -> [w592] mode=indexing
          shift-right: [w578] -> w555
          shift-left: w563 -> [w590]
          tunnel: [w577] -> w562 mode=indexing
          w580 = "Axis " ("string")
          # "Update Axes names"
          # "Update Graph Window Titles"
          n245 = Unbundle By Name(w592) -> ("Scan"=w579:string, "Scan Axis"=w584:string, "Step Axis"=w583:string)
          n246 = Concatenate Strings("Area Scan Routine " ("string"), w579) -> (w593:string)
          n247 = Concatenate Strings(w580, w584) -> (w581:string)
          n248 = Concatenate Strings(w580, w583) -> (w582:string)
          n249 = property class="VI"(reference=w591, error in=w590, "Front Panel.Title"=w593) -> (reference out=w589:refnum<vi>, error out=w588:errorcluster)
          n250 = Build Array(w581, w582, "Intensity" ("string")) -> (w585:string[])
          n251 = invoke class="VI" method="Ctrl Val.Set"(reference=w589, error in=w588, "Control Name"="Axes names" ("string"), "Value"=w585) -> (reference out=w577:refnum<vi>, error out=w578:errorcluster)  [unwired: 1 in, 3 out]
        }
        "3DGraphReferenceArray" <- w562
      }
      frame "Reset Area Scan Graph References" {
        w614 = 0  # No. Area Scans
        n252 = local read "3DGraphReferenceArray"() -> (w613:refnum<vi>[])
        n253 = for {
          tunnel: w613 -> [w625] mode=indexing
          tunnel: w612 -> [w622]
          tunnel: [w621] -> w604
          n254 = invoke class="VI" method="Abort VI"(reference=w625, error in=w622) -> (reference out=w624:refnum<vi>, error out=w623:errorcluster)  [unwired: 1 in, 1 out]
          n255 = invoke class="VI" method="FP.Close"(reference=w624, error in=w623) -> (error out=w621:errorcluster)  [unwired: 1 in, 2 out]
        }
        n256 = Unbundle By Name(w604) -> ("code"=w603:i32)
        n257 = case shown="1000" w603 {
          tunnel: w604 -> [w617 w619]
          tunnel: [w617 w618] -> w602
          frame 0, Default {
          }
          frame 1000 {
            n258 = call <vilib>:"Clear Errors.vi"("error in (no error)"=w619) -> ("error out"=w618:errorcluster)  [unwired: 1 in, 5 out]
          }
        }
        n259 = Array Size(array=w606) -> (size(s)=w605:i32)
        n260 = flat-sequence {
          tunnel: w602 -> [_]
          frame #0 {
            w620 = refnum<vi>[] []  # 3DGraphReferenceArray
            n261 = local write "3DGraphReferenceArray"(w620) -> ()
          }
        }
        n262 = Bundle By Name(cluster=T5 {"Message"="", "Message Data"=variant} ("Message Cluster"), "Message"="Update Area Scan Graph References", "Message Data"=w605) -> (w609:T5)
        n263 = Enqueue Element At Opposite End(queue=w608, element=w609, error in (no error)=w602) -> (error out=w607:errorcluster)  [unwired: 3 out]
      }
      frame "Update Area Scan Graph Data" {
        # "Set control values of area scan routine 3D windows and trigger to update data."
        n264 = local read "3DGraphReferenceArray"() -> (w632:refnum<vi>[])
        n265 = local read "Area Scan Routines"() -> (w626:T3)
        n266 = call "GetAreaScanAxesRanges.vi"("System no."=w628, "error in"=w630) -> ("Scan Ranges"=w627:T15, "error out"=w629:errorcluster)  [unwired: 16 out]
        n267 = for {
          shift-right: [w636] -> w631
          shift-left: w629 -> [w651]
          tunnel: w632 -> [w646] mode=indexing
          tunnel: w627 -> [w643]
          tunnel: w626 -> [w642] mode=indexing
          i -> [w650]
          n268 = Unbundle By Name(w642) -> ("Scan"=w641:string)
          n269 = for {
            tunnel: w641 -> [w656]
            tunnel: w643 -> [w657] mode=indexing
            tunnel: [w657] -> w645
            stop <- w658 stop-if-true
            n270 = Unbundle By Name(w657) -> ("Scan name"=w659:string)
            n271 = Equal?(x=w659, y=w656) -> (x = y?=w658:bool)
          }
          n272 = local read "Area Scan Data"() -> (w649:dbl[][][])
          n273 = invoke class="VI" method="Ctrl Val.Set"(reference=w646, error in=w651, "Control Name"="Area Scan Data", "Value"=w649) -> (reference out=w653:refnum<vi>, error out=w652:errorcluster)  [unwired: 1 in, 3 out]
          n274 = invoke class="VI" method="Ctrl Val.Set"(reference=w653, error in=w652, "Control Name"="Area Scan Data page", "Value"=w650) -> (reference out=w639:refnum<vi>, error out=w640:errorcluster)  [unwired: 1 in, 3 out]
          n275 = invoke class="VI" method="Ctrl Val.Set"(reference=w639, error in=w640, "Control Name"="Scan range" ("string"), "Value"=w645) -> (reference out=w637:refnum<vi>, error out=w638:errorcluster)  [unwired: 1 in, 3 out]
          n276 = invoke class="VI" method="Ctrl Val.Set"(reference=w637, error in=w638, "Control Name"="Update Data", "Value"=1) -> (error out=w636:errorcluster)  [unwired: 1 in, 4 out]
        }
      }
      frame "Update Scan Control Clusters" {
        # "Read all scan routine definitions from controller and update scan control clusters."
        n277 = call "GetGradientSearchNamesAndAxes.vi"("System no."=w660, "error in"=w665) -> ("Scan Name, Scan Axis, Step Axis"=w663:string[][], "error out"=w667:errorcluster)  [unwired: 16 out]
        n278 = call "GetAreaScanNamesAndAxes.vi"("System no."=w660, "error in"=w667) -> ("Scan Name, Scan Axis, Step Axis"=w678:string[][], "error out"=w666:errorcluster)  [unwired: 16 out]
        n279 = for {
          tunnel: w660 -> [w688]
          tunnel: w663 -> [w686] mode=indexing
          tunnel: [w687] -> w662 mode=indexing
          tunnel: "Gradient Scan Routines" -> [w685]
          tunnel: [w683] -> w661 mode=indexing
          i -> [w684]
          n280 = global read "Global2 (Array).vi" "System"() -> (w692:T13)
          n281 = Decrement(x=w688) -> (x-1=w691:i32)
          n282 = Index Array(array=w692, index=w691) -> (element=w690:T14)
          n283 = Unbundle By Name(w690) -> ("Controller name"=w689:T2)
          n284 = Index Array(array=w685, index=w684) -> (element=w682:T6)
          n285 = Index Array(array=w686) -> (element #1=w683:string, element #2=w681:string, element #3=w680:string)  [unwired: 3 in]
          n286 = Bundle By Name(cluster=w682, "Sys"=w688, "Controller"=w689, "Scan"=w683, "Scan Axis"=w681, "Step Axis"=w680) -> (w687:T6)
        }
        "Gradient Scan Names" <- w661
        n287 = for {
          tunnel: w660 -> [w709]
          tunnel: w678 -> [w707] mode=indexing
          tunnel: [w708] -> w677 mode=indexing
          tunnel: "Area Scan Routines" -> [w706]
          tunnel: [w704] -> w675 mode=indexing
          i -> [w705]
          n288 = global read "Global2 (Array).vi" "System"() -> (w713:T13)
          n289 = Decrement(x=w709) -> (x-1=w712:i32)
          n290 = Index Array(array=w713, index=w712) -> (element=w711:T14)
          n291 = Unbundle By Name(w711) -> ("Controller name"=w710:T2)
          n292 = Index Array(array=w706, index=w705) -> (element=w703:T7)
          n293 = Index Array(array=w707) -> (element #1=w704:string, element #2=w702:string, element #3=w701:string)  [unwired: 3 in]
          n294 = Bundle By Name(cluster=w703, "Sys"=w709, "Controller"=w710, "Scan"=w704, "Scan Axis"=w702, "Step Axis"=w701) -> (w708:T7)
        }
        n295 = Array Size(array=w662) -> (size(s)=w679:i32)
        n296 = local write "Gradient Scan Routines"(w662) -> ()
        n297 = Array Size(array=w677) -> (size(s)=w673:i32)
        n298 = local write "Area Scan Routines"(w677) -> ()
        n299 = Array Size(array="Area Scan Routines") -> (size(s)=w672:i32)
        n300 = property on="Area Scan Routines" class="Arr"("Number of Rows"=w673) -> ()  [unwired: 2 in, 2 out]
        n301 = property on="Gradient Scan Routines" class="Arr"("Number of Rows"=w679) -> ()  [unwired: 2 in, 2 out]
        n302 = local read "Area Scan Data"() -> (w668:dbl[][][])
        n303 = Subtract(x=w673, y=w672) -> (x-y=w669:i32)
        n304 = Greater?(x=w673, y=w672) -> (0:w671:bool)
        n305 = case shown="True" w671 {
          tunnel: w668 -> [w693 w695]
          tunnel: [w693 w696] -> w670
          tunnel: w669 -> [_ w697]
          frame False {
          }
          frame True {
            n306 = for {
              N: w697 -> [_]
              shift-right: [w698] -> w696
              shift-left: w695 -> [w700]
              tunnel: dbl[][] [[0.0]] ("Area Scan Data") -> [w699]
              n307 = Build Array (concatenate)(w700, w699) -> (w698:dbl[][][])
            }
          }
        }
        n308 = local write "Area Scan Data"(w670) -> ()
      }
      frame "Update Display" {
        w746 = string[] []
        # "Query status, center position and radius of gradient scan routines.\nQuery position of all axes.\nQuery scan routine results.\nQuery calculated value of analog input.\n\nPut all those values in queues so that all of the sub VIs can work with the data."
        n309 = Array Size(array=w729) -> (size(s)=w735:i32)
        n310 = Array Size(array=w718) -> (size(s)=w719:i32)
        n311 = Greater Than 0?(x=w719) -> (x > 0?=w717:bool)
        n312 = local read "Gradient Scan Routines"() -> (w714:T4)
        n313 = Greater?(x=w735, y=w733) -> (0:w736:bool)
        n314 = case shown="True" w717 {
          tunnel: w750 -> [w774 w779]
          tunnel: [w774 w778] -> w749
          tunnel: [bool[] [] w777] -> w740
          tunnel: w731 -> [_ w776]
          tunnel: w718 -> [_ w775]
          frame False {
          }
          frame True {
            n315 = call "FRP?.vi"("System no."=w776, "Routines to query"=w775, "error in"=w779) -> ("Status"=w780:i32[], "error out"=w778:errorcluster)  [unwired: 1 in, 14 out]
            n316 = Equal?(x=w780, y=2 ("Numeric")) -> (x = y?=w777:bool[])
          }
        }
        n317 = case shown="True" w736 {
          tunnel: w735 -> [_ w785]
          tunnel: [w782 w785] -> w734
          tunnel: w733 -> [w782 w784]
          tunnel: w732 -> [_ w788]
          frame False {
          }
          frame True {
            n318 = Subtract(x=w785, y=w784) -> (x-y=w783:i32)
            n319 = Bundle By Name(cluster=T5 {"Message"="Update Area Scan Graph References", "Message Data"=variant} ("Message Cluster"), "Message Data"=w783) -> (w786:T5)
            n320 = Enqueue Element At Opposite End(queue=w788, element=w786) -> ()  [unwired: 1 in, 4 out]
          }
        }
        n321 = for {
          tunnel: w740 -> [w798] mode=indexing
          tunnel: [w799] -> w751 mode=indexing
          shift-right: [w793] -> w742
          shift-left: w746 -> [w794]
          shift-right: [w790] -> w741
          shift-left: w746 -> [w791]
          tunnel: w714 -> [w789]
          i -> [w797]
          n322 = Index Array(array=w789, index=w797) -> (element=w796:T6)
          n323 = Bundle By Name(cluster=w796, "Running"=w798) -> (w799:T6)
          n324 = Unbundle By Name(w796) -> ("Scan Axis"=w795:string, "Step Axis"=w792:string)
          n325 = Build Array (concatenate)(w794, w795) -> (w793:string[])
          n326 = Build Array (concatenate)(w791, w792) -> (w790:string[])
        }
        n327 = call "POS?.vi"("System no."=w731, "All axes?"=TRUE, "error in"=w749) -> ("Position"=w758:dbl[], "error out"=w747:errorcluster)  [unwired: 2 in, 13 out]
        n328 = To Variant(anything=w758) -> (Variant=w756:variant)
        n329 = Bundle By Name(cluster=T5 {"Message"="GraphData", "Message Data"=variant} ("Message Cluster"), "Message Data"=w756) -> (w759:T5)
        n330 = local write "Gradient Scan Routines"(w751) -> ()
        n331 = Lossy Enqueue Element(queue=w760, element=w759, error in (no error)=w747) -> (error out=w745:errorcluster)  [unwired: 3 out]
        n332 = case shown="True" w717 {
          tunnel: w745 -> [w762 w772]
          tunnel: [w762 w771] -> w744
          tunnel: w742 -> [_ w770]
          tunnel: w741 -> [_ w769]
          tunnel: w740 -> [_ w768]
          tunnel: [w761 w767] -> w739
          tunnel: [w761 w766] -> w738
          tunnel: [w761 w765] -> w737
          tunnel: w731 -> [_ w764]
          tunnel: w718 -> [_ w763]
          frame False {
            w761 = dbl[] [] ("Step Axes Center")
          }
          frame True {
            n333 = call "GetScanCenterAndRadius.vi"("System no."=w764, "Gradient Scan Names"=w763, "Scan Axes"=w770, "Step Axes"=w769, "Scan Routine Running?"=w768, "error in"=w772) -> ("Scan Axes Center"=w767:dbl[], "Step Axes Center"=w766:dbl[], "Current Radius"=w765:dbl[], "error out"=w771:errorcluster)  [unwired: 10 out]
          }
        }
        n334 = Bundle(cluster=T10 {"Gradient Scan Names"=[], "Dither Radius"=[], "Scan axis center"=[], "Step axis center"=[]}, "Gradient Scan Names"=w718, "Dither Radius"=w737, "Scan axis center"=w739, "Step axis center"=w738) -> (w755:T10)
        n335 = Bundle By Name(cluster=T5 {"Message"="", "Message Data"=variant} ("Message Cluster"), "Message Data"=w755) -> (w757:T5)
        n336 = Lossy Enqueue Element(queue=w721, element=w757, error in (no error)=w744) -> (error out=w730:errorcluster)  [unwired: 3 out]
        n337 = Build Array (concatenate)(w718, w729) -> (w728:string[])
        n338 = call "QueryFastRoutineResults.vi"("System No."=w731, "Fast Routine Names"=w728, "No. Routines to query at once"=1 ("No. Scans to query at once"), "error in"=w730) -> ("Routine Results"=w727:T16, "error out"=w725:errorcluster)  [unwired: 14 out]
        n339 = Bundle By Name(cluster=T5 {"Message"="", "Message Data"=variant} ("Message Cluster"), "Message Data"=w727) -> (w722:T5)
        n340 = Lossy Enqueue Element(queue=w726, element=w722, error in (no error)=w725) -> (error out=w724:errorcluster)  [unwired: 3 out]
        n341 = call "TCI?.vi"("System no."=w731, "Board"="Analog Input", "error in"=w724) -> ("Calculated analog value"=→"Waveform Chart" →"Analog value":dbl, "error out"=w753:errorcluster)  [unwired: 15 out]
      }
      frame "MVR" {
        # "Move axis relatively to it's current position."
        n342 = Variant To Data(error in=w815, type=T11 {"Axis"="", "Target"=0.0, "System no."=0}, Variant=w813) -> (data=w812:T11, error out=w814:errorcluster)
        n343 = local read "Gradient Scan Routines"() -> (w802:T4)
        n344 = Unbundle By Name(w812) -> ("System no."=w800:i32, "Axis"=w807:string, "Target"=w803:dbl)
        n345 = for {
          tunnel: w807 -> [w857]
          tunnel: [w855] -> w806
          tunnel: [w854] -> w805
          tunnel: [w853] -> w804
          tunnel: w802 -> [w851] mode=indexing
          stop <- w855 stop-if-true
          n346 = Unbundle By Name(w851) -> ("Scan Axis"=w850:string, "Step Axis"=w849:string, "Running"=w848:bool, "Scan"=w854:string)
          n347 = Equal?(x=w857, y=w850) -> (x = y?=w853:bool)
          n348 = Equal?(x=w857, y=w849) -> (x = y?=w852:bool)
          n349 = Or(x=w853, y=w852) -> (x .or. y?=w856:bool)
          n350 = And(x=w856, y=w848) -> (x .and. y?=w855:bool)
        }
        n351 = Build Array(w807) -> (w811:string[])
        n352 = case shown="True" w806 {
          tunnel: [w823 w837] -> w817
          tunnel: w814 -> [w822 w839]
          tunnel: w811 -> [w821 _]
          tunnel: w800 -> [w820 w833]
          tunnel: w805 -> [_ w838]
          tunnel: w804 -> [_ w836]
          tunnel: w803 -> [w818 w832]
          frame False {
            # "Use normal MVR command if axis is not part of a running scan routine."
            n353 = Build Array(w818) -> (w819:dbl[])
            n354 = call "MVR.vi"("System no."=w820, "Axes to move"=w821, "Position values"=w819, "error in"=w822) -> ("error out"=w823:errorcluster)  [unwired: 1 in, 14 out]
          }
          frame True {
            # "Use FGC? + FGC while scan routine is running."
            n355 = Build Array(w838) -> (w824:string[])
            n356 = call "FGC?.vi"("System no."=w833, "Routine name"=w824, "error in"=w839) -> ("Scan axis center"=w831:dbl[], "Step axis center"=w830:dbl[], "Queried routine name out"=w835:string[], "error out"=w825:errorcluster)  [unwired: 1 in, 12 out]
            n357 = Index Array(array=w831) -> (element=w829:dbl)  [unwired: 1 in]
            n358 = Index Array(array=w830) -> (element=w828:dbl)  [unwired: 1 in]
            n359 = case shown="True" w836 {
              tunnel: w832 -> [w843 w847]
              tunnel: w829 -> [w840 w846]
              tunnel: w828 -> [w842 w844]
              tunnel: [w840 w845] -> w827
              tunnel: [w841 w844] -> w826
              frame False {
                # "Move Step Axis"
                n360 = Add(x=w843, y=w842) -> (x+y=w841:dbl)
              }
              frame True {
                # "Move Scan Axis"
                n361 = Add(x=w847, y=w846) -> (x+y=w845:dbl)
              }
            }
            n362 = Index Array(array=w835) -> (element=w834:string)  [unwired: 1 in]
            n363 = call "FGC.vi"("System no."=w833, "Routine name"=w834, "Scan axis value"=w827, "Step axis value"=w826, "error in"=w825) -> ("error out"=w837:errorcluster)  [unwired: 2 in, 12 out]
          }
        }
      }
      frame "MOV" {
        w858 = FALSE  # All axes?
        # "Move axis absolut"
        n364 = Variant To Data(error in=w873, type=T11 {"Axis"="", "Target"=0.0, "System no."=0}, Variant=w871) -> (data=w870:T11, error out=w872:errorcluster)
        n365 = Unbundle By Name(w870) -> ("System no."=w860:i32, "Axis"=w866:string, "Target"=w865:dbl)
        n366 = Build Array(w866) -> (w859:string[])
        n367 = Build Array(w865) -> (w863:dbl[])
        n368 = call "MOV.vi"("System no."=w860, "Axes to move"=w859, "Position values"=w863, "error in"=w872) -> ("error out"=w862:errorcluster)  [unwired: 1 in, 14 out]
        n369 = call "General wait for movement to stop.vi"("System no."=w860, "Axes to wait for"=w859, "All axes?"=w858, "error in"=w862) -> ("error out"=w861:errorcluster)  [unwired: 4 in, 11 out]
      }
      frame "Send String" {
        w881 = TRUE  # Attach termination char.?
        n370 = Variant To Data(error in=w887, type=T12 {"String to send"="", "System no."=0}, Variant=w886) -> (data=w885:T12, error out=w880:errorcluster)
        n371 = Unbundle By Name(w885) -> ("System no."=w875:i32, "String to send"=w878:string)
        n372 = call "PI Send String.vi"("System no."=w875, "String to send"=w878, "Attach termination char.?"=w881, "error in"=w880) -> ("error out"=w877:errorcluster)  [unwired: 15 out]
        n373 = call "ERR?.vi"("System no."=w875, "error in"=w877) -> ("error out"=w876:errorcluster)  [unwired: 17 out]
      }
      frame "Start GS Routines" {
        # "Start selected gradient scan routines."
        n374 = local read "Gradient Scan Routines"() -> (w897:T4)
        n375 = for {
          shift-right: [w910] -> w895
          shift-left: string[] [] -> [w911]
          tunnel: w897 -> [w909] mode=indexing
          n376 = Unbundle By Name(w909) -> ("Enable"=w908:bool, "Scan"=w912:string)
          n377 = case shown="True" w908 {
            tunnel: w912 -> [_ w914]
            tunnel: w911 -> [w913 w916]
            tunnel: [w913 w915] -> w910
            frame False {
            }
            frame True {
              n378 = Build Array (concatenate)(w916, w914) -> (w915:string[])
            }
          }
        }
        n379 = Array Size(array=w895) -> (size(s)=w894:i32)
        n380 = Greater Than 0?(x=w894) -> (x > 0?=w893:bool)
        n381 = case shown="True" w893 {
          tunnel: [w903 w907] -> w892
          tunnel: w902 -> [w903 w906]
          tunnel: w898 -> [_ w905]
          tunnel: w895 -> [_ w904]
          frame False {
          }
          frame True {
            n382 = call "FRS.vi"("System no."=w905, "Routines to start"=w904, "error in"=w906) -> ("error out"=w907:errorcluster)  [unwired: 16 out]
          }
        }
        n383 = Enqueue Element At Opposite End(queue=w890, element=T5 {"Message"="Show ScanResults Window", "Message Data"=variant} ("Message Cluster"), error in (no error)=w892) -> (error out=w891:errorcluster)  [unwired: 3 out]
      }
      frame "Show ScanResults Window" {
        # "Open front panel of scan results window if it is not opened at the moment."
        n384 = vi-ref "RoutineResults.vi"() -> (w922:refnum<vi>)
        n385 = property class="VI"(reference=w922) -> (error out=w923:errorcluster, "Path"=w924:path)  [unwired: 1 in, 1 out]
        n386 = Open VI Reference(vi path=w924, error in (no error)=w923) -> (vi reference=w919:refnum<vi>, error out=w921:errorcluster)  [unwired: 1 in, 3 out]
        n387 = property class="VI"(reference=w919, error in=w921) -> (reference out=w918:refnum<vi>, error out=w920:errorcluster, "Front Panel.Open"=w917:bool)
        n388 = case shown="True" w917 {
          tunnel: w920 -> [w932 _]
          tunnel: w918 -> [w931 _]
          frame False {
            n389 = property class="VI"(reference=w931, error in=w932, "Front Panel.Open"=TRUE ("Front Panel Window:Open")) -> (reference out=w933:refnum<vi>, error out=w934:errorcluster)
            n390 = invoke class="VI" method="Run VI"(reference=w933, error in=w934, "Wait until done"=FALSE ("Wait Until Done"), "Auto Dispose Ref"=TRUE ("Front Panel Window:Open")) -> ()  [unwired: 1 in, 5 out]
          }
          frame True {
          }
        }
      }
      frame "Start AS Routines" {
        # "Set timeout to infinity, so that the qeue doesn't\nget full while aquiring data from data recorder."
        # "Indicate that scan is running"
        n391 = flat-sequence {
          tunnel: w961 -> [_]
          tunnel: [w1037] -> w965
          tunnel: w965 -> [w1038]
          tunnel: [w1038] -> w944
          frame #0 {
            n392 = local read "Event timeout"() -> (w1037:i32)
          }
          frame #1 {
            n393 = local write "Event timeout"(-1) -> ()
          }
        }
        n394 = Enqueue Element At Opposite End(queue=w960, element=T5 {"Message"="Update Area Scan Graph Data", "Message Data"=variant} ("Message Cluster"), error in (no error)=w961) -> (error out=w959:errorcluster)  [unwired: 3 out]
        n395 = local read "Area Scan Routines"() -> (w946:T3)
        n396 = Variant To Data(error in=w959, type=T7 {"Sys"=1, "Controller"=enum."None", "Scan"="", "Scan Axis"="", "Step Axis"="", "Running"=FALSE, "Record\ndata"=FALSE, "Show Graph"=FALSE, "Save Data"=FALSE, "Start Scan"=FALSE} ("GradientScans"), Variant=w958) -> (data=w945:T7, error out=w940:errorcluster)
        n397 = Unbundle By Name(w945) -> ("Sys"=w941:i32, "Record\ndata"=w947:bool, "Scan"=w957:string, "Scan Axis"=w956:string, "Step Axis"=w955:string)
        n398 = for {
          tunnel: w946 -> [w982] mode=indexing
          tunnel: w957 -> [w983]
          tunnel: [w979] -> w937
          i -> [w977]
          stop <- w980 stop-if-true
          # "Start selected area scan routine."
          n399 = Unbundle By Name(w982) -> ("Scan"=w981:string)
          n400 = Equal?(x=w983, y=w981) -> (x = y?=w980:bool)
          n401 = Select(t=w977, s=w980, f=-1) -> (s? t:f=w979:i32)
        }
        n402 = local read "Area Scan Data"() -> (w962:dbl[][][])
        n403 = case shown="True" w947 {
          tunnel: w957 -> [w988 w1000]
          tunnel: w956 -> [_ w1021]
          tunnel: w955 -> [_ w1020]
          tunnel: w940 -> [w990 w1003]
          tunnel: [w986 w1022] -> w939
          tunnel: w941 -> [w989 w1002]
          tunnel: [w987 w1008] -> w966
          tunnel: w962 -> [w987 w1015]
          tunnel: w937 -> [_ w1006]
          tunnel: w944 -> [w984 w1007]
          tunnel: [w984 w1007] -> w943
          frame False {
            # "Start area scan routine without recording data."
            # "Wait for scan to be finished"
            # "Start scan routine"
            n404 = Build Array(w988) -> (w985:string[])
            n405 = call "FRS.vi"("System no."=w989, "Routines to start"=w985, "error in"=w990) -> ("error out"=w993:errorcluster)  [unwired: 16 out]
            n406 = Array Size(array=w985) -> (size(s)=w994:i32)
            n407 = Initialize Array(0 ("element"), w994) -> (w996:i32[])
            n408 = call "WaitForFRPQuery.vi"("System no."=w989, "Routines to query"=w985, "Query all routines?"=FALSE ("All routines?"), "Option"=w996, "error in"=w993, "Timeout / ms"=u32 60000) -> ("error out"=w986:errorcluster)  [unwired: 1 in, 12 out]
          }
          frame True {
            w997 = 150  # Record Option  for Optical Channel
            # "Record scan data if selected. This may take some time..."
            # "Read Data from\nData Recorder"
            # "Wait for scan to be finished"
            # "Start scan routine"
            # "Configure Data Recorder"
            n409 = call "GetFastAlignmentInputID.vi"("System no."=w1002, "Scan Name in"=w1000, "Fast Routine type"=enum16{"FDG", "FDR"}."FDR", "error in"=w1003) -> ("Analog channel out"=w999:i32, "error out"=w1001:errorcluster)  [unwired: 14 out]
            n410 = Build Array(w1021, w1020) -> (w1031:string[])
            n411 = Increment(x=w1006) -> (x+1=w1005:i32)
            n412 = call "ConfigureDataRecorder.vi"("System no."=w1002, "Axes"=w1031, "Analog Input"=w999, "Record Option for Optical Channel"=w997, "error in (no error)"=w1001) -> ("Rec. table IDs Out"=w1026:i32[], "error out"=w1032:errorcluster)  [unwired: 1 in, 12 out]
            n413 = Build Array(w1000) -> (w1030:string[])
            n414 = Array Size(array=w1015) -> (size(s)=w1018:i32[])
            n415 = call "FRS.vi"("System no."=w1002, "Routines to start"=w1030, "error in"=w1032) -> ("error out"=w1033:errorcluster)  [unwired: 16 out]
            n416 = Index Array(array=w1018, index=0) -> (element=w1014:i32)
            n417 = Array Size(array=w1030) -> (size(s)=w1034:i32)
            n418 = Initialize Array(0 ("element"), w1034) -> (w1036:i32[])
            n419 = Array Subset(array=w1015, index (dim 0)=0, length (dim 0)=w1006) -> (w1011:dbl[][][])  [unwired: 4 in]
            n420 = call "WaitForFRPQuery.vi"("System no."=w1002, "Routines to query"=w1030, "Query all routines?"=FALSE ("All routines?"), "Option"=w1036, "error in"=w1033, "Timeout / ms"=u32 60000) -> ("error out"=w1027:errorcluster)  [unwired: 1 in, 12 out]
            n421 = call "DRL?.vi"("System no."=w1002, "Rec. table to query"=w1026, "With Rec. table IDs?"=TRUE, "error in"=w1027) -> ("No. of rec. values"=w1024:i32[], "error out"=w1028:errorcluster)  [unwired: 14 out]
            n422 = Increment(x=w1006) -> (x+1=w1013:i32)
            n423 = Subtract(x=w1014, y=w1005) -> (x-y=w1012:i32)
            n424 = Index Array(array=w1024, index=0) -> (element=w1004:i32)
            n425 = Array Subset(array=w1015, index (dim 0)=w1013, length (dim 0)=w1012) -> (w1009:dbl[][][])  [unwired: 4 in]
            n426 = call "DRR?.vi"("System no."=w1002, "Rec. table IDs"=w1026, "error in"=w1028, "N"=w1004, "Nmax"=w1004) -> ("Data"=w1010:dbl[][], "error out"=w1022:errorcluster)  [unwired: 3 in, 10 out]
            n427 = Build Array (concatenate)(w1011, w1010, w1009) -> (w1008:dbl[][][])
          }
        }
        "Area Scan Data" <- w966
        n428 = Bundle By Name(cluster=w945, "Running"=TRUE ("With Rec. table IDs?")) -> (w953:T7)
        n429 = Replace Array Subset(array=w946, new element=w953, index=w937) -> (w952:T3)
        n430 = local write "Area Scan Routines"(w952) -> ()
        n431 = local write "Event timeout"(w943) -> ()
        n432 = Bundle By Name(cluster=w945, "Running"=FALSE ("With Rec. table IDs?")) -> (w949:T7)
        n433 = flat-sequence {
          tunnel: w946 -> [w976]
          tunnel: w937 -> [w975]
          tunnel: w949 -> [w974]
          tunnel: w939 -> [w971]
          tunnel: w942 -> [w970]
          tunnel: [w969] -> w938
          frame #0 {
            # "Trigger event loop to get out\nof the infinity timeout."
            n434 = Replace Array Subset(array=w976, new element=w974, index=w975) -> (w973:T3)
            n435 = Generate User Event(user event=w970, event data cluster=cluster{bool} {TRUE} ("event data"), error in=w971) -> (error out=w969:errorcluster)  [unwired: 1 in, 1 out]
            n436 = local write "Area Scan Routines"(w973) -> ()
          }
        }
      }
      frame "Stop GS Routines" {
        # "Stop all gradient scan routines that are running."
        n437 = local read "Gradient Scan Routines"() -> (w1043:T4)
        n438 = for {
          shift-right: [w1061] -> w1049
          shift-left: string[] [] -> [w1062]
          tunnel: w1043 -> [w1060] mode=indexing
          n439 = Unbundle By Name(w1060) -> ("Running"=w1059:bool, "Scan"=w1063:string)
          n440 = case shown="False" w1059 {
            tunnel: w1063 -> [_ w1065]
            tunnel: w1062 -> [w1064 w1067]
            tunnel: [w1064 w1066] -> w1061
            frame False {
            }
            frame True {
              n441 = Build Array (concatenate)(w1067, w1065) -> (w1066:string[])
            }
          }
        }
        n442 = Array Size(array=w1049) -> (size(s)=w1041:i32)
        n443 = Greater Than 0?(x=w1041) -> (x > 0?=w1040:bool)
        n444 = Initialize Array(0 ("dimension size"), w1041) -> (w1047:i32[])
        n445 = case shown="True" w1040 {
          tunnel: [w1053 w1058] -> w1052
          tunnel: w1051 -> [w1053 w1057]
          tunnel: w1049 -> [_ w1056]
          tunnel: w1047 -> [_ w1055]
          tunnel: w1044 -> [_ w1054]
          frame False {
          }
          frame True {
            n446 = call "FRP.vi"("System no."=w1054, "Routinename"=w1056, "Option"=w1055, "error in"=w1057) -> ("error out"=w1058:errorcluster)  [unwired: 15 out]
          }
        }
      }
      frame "Exit" {
        w1071 = T5 {"Message"="Exit", "Message Data"=variant} ("element")
        # "Send \"Exit\" to all queues to shut down safely."
        # "close GS Graph Windows"
        n447 = local read "3DGraphReferenceArray"() -> (w1069:refnum<vi>[])
        n448 = local write "Status Message"("Shutting down..." ("L10n_Stop Pressed")) -> ()
        n449 = Enqueue Element At Opposite End(queue=w1083, element=w1071, error in (no error)=w1082) -> (queue out=w1081:refnum<queue>, error out=w1080:errorcluster)  [unwired: 2 out]
        n450 = for {
          tunnel: w1069 -> [w1089] mode=indexing
          n451 = invoke class="VI" method="Abort VI"(reference=w1089) -> (reference out=w1088:refnum<vi>, error out=w1087:errorcluster)  [unwired: 2 in, 1 out]
          n452 = invoke class="VI" method="FP.Close"(reference=w1088, error in=w1087) -> ()  [unwired: 1 in, 3 out]
        }
        n453 = call "Time Delay"("error in (no error)"=w1080) -> ("error out"=w1079:errorcluster)  [unwired: 1 in, 9 out]
        n454 = Release Queue(queue=w1081, error in (no error)=w1079) -> (error out=w1074:errorcluster)  [unwired: 3 out]
        n455 = Lossy Enqueue Element(queue=w1073, element=w1071, error in (no error)=w1074) -> (error out=w1072:errorcluster)  [unwired: 3 out]
        n456 = Lossy Enqueue Element(queue=w1070, element=w1071, error in (no error)=w1072) -> (error out=w1068:errorcluster)  [unwired: 3 out]
        n457 = flat-sequence {
          tunnel: w1068 -> [_]
          frame #0 {
            n458 = local write "Status Message"("") -> ()
          }
        }
      }
      frame Default {
      }
    }
    n459 = Unbundle By Name(w235) -> ("status"=w233:bool, "source"=w234:string)
    n460 = case shown="True" w233 {
      selector: w233 -> [_ w255]
      tunnel: w234 -> [_ w257]
      frame False {
      }
      frame True {
        n461 = Concatenate Strings("Error in\n", w257) -> (w256:string)
        n462 = local write "Status Message"(w256) -> ()
        n463 = property on="Clear Error" class="Bool"("Visible"=w255) -> ()  [unwired: 2 in, 2 out]
      }
    }
  }
  n464 = Merge Errors(w18, w17) -> (w16:errorcluster)
  n465 = call <vilib>:"Simple Error Handler.vi"("error in (no error)"=w16) -> ()  [unwired: 1 in, 8 out]
